vi "Get Server Alias from LabVIEW Server ID.vi"(7 "LabVIEW Server ID":string, 10 "Error In":errorcluster) -> (2 "Error Out":errorcluster, 3 "Server Alias":string)   [LabVIEW 2013, in "TS.lvlib"]
uses:
  TS.lvlib
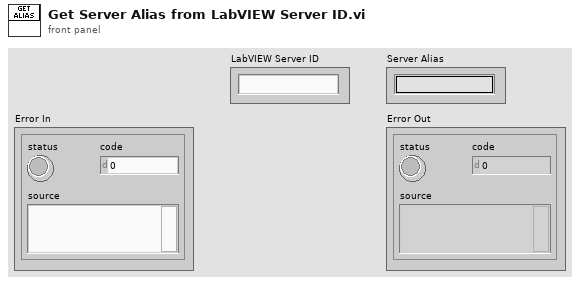
[diagram p1: front panel]
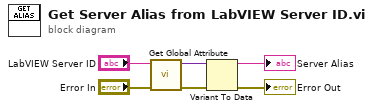
[diagram p0: block diagram]
diagram:
  n1 = call "Get Global Attribute.vi"("Error In"="Error In", "Name"="LabVIEW Server ID") -> ("Error Out"=w6:errorcluster, "Value"=w5:variant)  [unwired: 7 in, 1 out]
  n2 = Variant To Data(error in=w6, Variant=w5) -> (data=→"Server Alias":string, error out=→"Error Out":errorcluster)  [unwired: 1 in]
